vi "get_switch.vi"(8 "error in (no error)":errorcluster, 10 "channel":u16, 11 "Agilent 34980A in":refnum<class "Agilent 34980A.lvclass">) -> (0 "error out":errorcluster, 1 "String":string, 2 "actual switch state":bool, 3 "Agilent 34980A out":refnum<class "Agilent 34980A.lvclass">)   [LabVIEW 2017, in "Agilent 34980A.lvclass"]
doc: "get state of a specific switch channel from the actual instrument"
uses:
  Agilent 34980A.lvclass
  instrument.lvclass
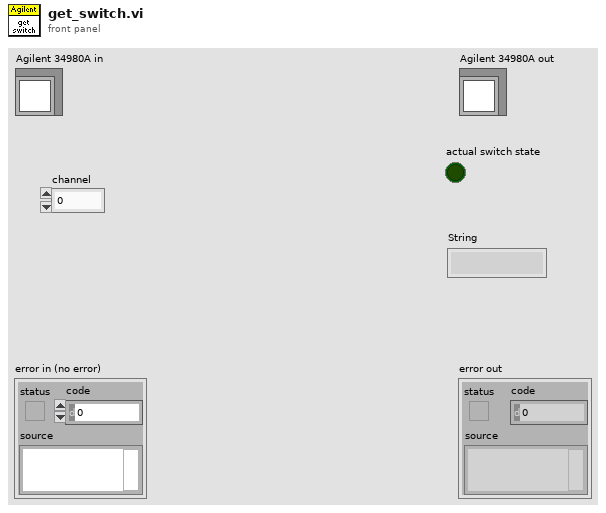
[diagram p1: front panel]
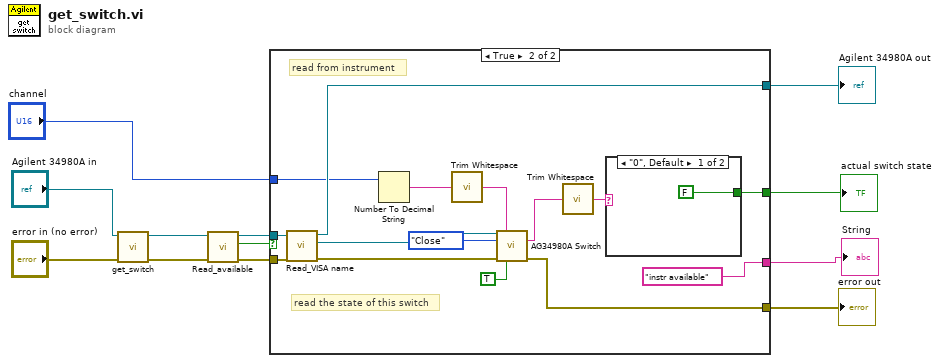
[diagram p0: block diagram]
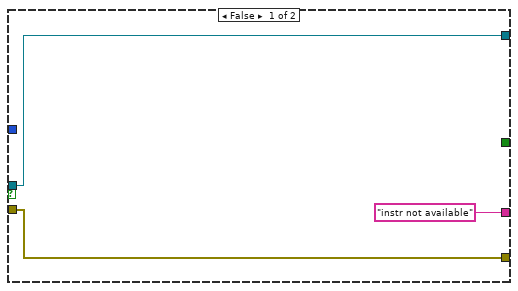
[diagram p2: hidden frame]
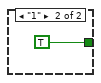
[diagram p3: hidden frame]
diagram:
  n1 = call-parent "get_switch.vi"("error in (no error)"="error in (no error)", "instrument in"="Agilent 34980A in") -> ("error out"=w6:errorcluster, "instrument out"=w7:refnum<class "Agilent 34980A.lvclass">)  [unwired: 6 in, 2 out]
  n2 = call-dynamic "Read_available.vi"("error in (no error)"=w6, "instrument in"=w7) -> ("error out"=w9:errorcluster, "available?"=w8:bool, "instrument out"=w10:refnum<class "Agilent 34980A.lvclass">)  [unwired: 7 in]
  n3 = case shown="True" w8 {
    tunnel: [w15 w28] -> w4
    tunnel: [w14 w26] -> w3
    tunnel: "channel" -> [_ w21]
    tunnel: w10 -> [w15 w23]
    tunnel: w9 -> [w14 w22]
    tunnel: [_ w17] -> w2
    tunnel: ["instr not available" "instr available"] -> w1
    frame False {
    }
    frame True {
      # "read from instrument"
      # "read the state of this switch"
      n4 = call-dynamic "Read_VISA name.vi"("error in (no error)"=w22, "instrument in"=w23) -> ("error out"=w27:errorcluster, "VISA resource name"=w30:refnum<visa-resource-name>, "instrument out"=w28:refnum<class "Agilent 34980A.lvclass">)  [unwired: 7 in]
      n5 = Number To Decimal String(number=w21) -> (decimal integer string=w20:string)  [unwired: 1 in]
      n6 = call <vilib>:"Trim Whitespace.vi"("string"=w20) -> ("trimmed string"=w24:string)  [unwired: 1 in]
      n7 = call "AG34980A Switch.vi"("VISA resource name"=w30, "Channel List"=w24, "Open/Close (0:Close)"=enum16{"Close", "Open"}."Close", "error in (no error)"=w27, "Set/Check (F:Set)"=TRUE) -> ("Channel State?"=w18:string, "error out"=w26:errorcluster)  [unwired: 8 in, 1 out]
      n8 = call <vilib>:"Trim Whitespace.vi"("string"=w18) -> ("trimmed string"=w19:string)  [unwired: 1 in]
      n9 = case shown="\"0\", Default" w19 {
        tunnel: [FALSE TRUE] -> w17
        frame "0", Default {
        }
        frame "1" {
        }
      }
    }
  }
  "error out" <- w3
  "Agilent 34980A out" <- w4
  "actual switch state" <- w2
  "String" <- w1
